vi "MixedInstrumentReservation_CallCreateSessions_OnlySpecifiedInstrumentSessionsCreated.vi"(8 "error in":errorcluster) -> (0 "error out":errorcluster, 2 "result":string, 3 "pass":bool)   [LabVIEW 2020, in "MeasurementServerTests.lvlib"]
uses:
  MeasurementServerTests.lvlib
  da6ffb6f-c1c9-4957-84dd-e9228483c454.vi
  ffc64c76-1568-41a3-8328-b9126ac9a28d.vi
  Helpers/Fake Instrument/Fake Instrument.lvclass
  \\tsclient\C/dev/measurementlink-labview/Source/Runtime/MeasurementLink Instrument/IInstrument/IInstrument.lvclass
  Runtime/MeasurementLink Session Management/Session Reservation/Create Sessions Impl.vi
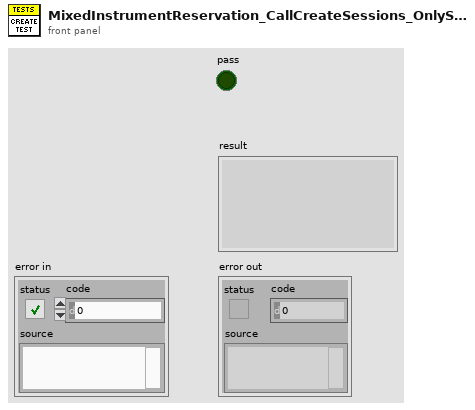
[diagram p1: front panel]
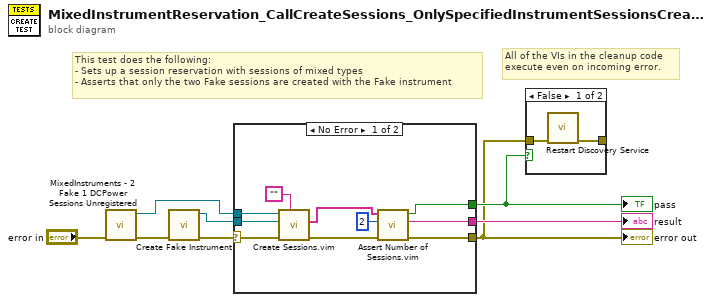
[diagram p0: block diagram]
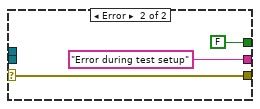
[diagram p2: hidden frame]
diagram:
  # "All of the VIs in the cleanup code\nexecute even on incoming error."
  # "This test does the following:\n- Sets up a session reservation with sessions of mixed types\n- Asserts that only the two Fake sessions are created with the Fake instrument"
  n1 = call "MixedInstruments - 2 Fake 1 DCPower Sessions Unregistered.vi"("error in (no error)"="error in") -> ("error out"=w2:errorcluster, "Session Reservation out"=w1:refnum<class "Session Reservation.lvclass">)  [unwired: 9 in]
  n2 = call "Create Fake Instrument.vi"("error in"=w2) -> ("error out"=w5:errorcluster, "fake instrument out"=w4:refnum<class "Fake Instrument.lvclass">)  [unwired: 9 in]
  n3 = case shown="No Error" w5 {
    selector: w5 -> [w16 w19]
    tunnel: [w11 w19] -> w6
    tunnel: [w9 FALSE] -> w7
    tunnel: [w10 "Error during test setup" ("f")] -> w8
    tunnel: w4 -> [w18 _]
    tunnel: w1 -> [w17 _]
    frame No Error {
      n4 = call "Create Sessions.vim"("session type"="", "error in"=w16, "instrument"=w18, "session reservation in"=w17) -> ("error out"=w15:errorcluster, "sessions"=w13:string[])  [unwired: 4 in, 2 out]
      n5 = call "Assert Number of Sessions.vim"("error in"=w15, "expected number of sessions"=2, "sessions"=w13) -> ("error out"=w11:errorcluster, "result"=w10:string, "pass"=w9:bool)  [unwired: 6 in]
    }
    frame Error {
    }
  }
  "error out" <- w6
  "pass" <- w7
  "result" <- w8
  n6 = case shown="False" w7 {
    tunnel: w6 -> [w23 _]
    tunnel: [w22 _] -> _
    frame False {
      n7 = call "Restart Discovery Service.vi"("error in"=w23) -> ("error out"=w22:errorcluster)  [unwired: 10 in]
    }
    frame True {
    }
  }
